vi "SetAttributeViString_SA-Gating_Sweep.vi"(7 "AttributeValue":string, 8 "error in (no error)":errorcluster {"code" format="%.0x"}, 9 "AttributeID":u32(ring)=1250201 items=["ACTIVE_MARKER"=1250201, "DISPLAY_TEXT"=1150119, "INPUT_RF_CORRECTION_COMMENT"=1150737, "INPUT_RF_CORRECTION_DESCRIPTION"=1150738, "IVILXISYNC_ARM_SOURCE_EVENTID"=1950012, "IVILXISYNC_ARM_SOURCE_FILTER"=1950013, "IVILXISYNC_EVENT_DESTINATION_PATH"=1950029, "IVILXISYNC_EVENT_SOURCE"=1950032, "IVILXISYNC_TRIGGER_SOURCE_EVENTID"=1950026, "IVILXISYNC_TRIGGER_SOURCE_FILTER"=1950027, "IVILXISYNC_TRIGGER_SOURCE"=1950022, "MARKER_TRACE"=1250209, "SA_ACP_DISPLAY_TEXT"=1150150, "SA_BURSTPOWER_DISPLAY_TEXT"=1150213, "SA_CHANNELPOWER_DISPLAY_TEXT"=1150305, "SA_LIMIT_COMMENT"=1150618, "SA_OCCUPIEDBANDWIDTH_DISPLAY_TEXT"=1150311, "SA_POWERSTATISTICS_DISPLAY_TEXT"=1150339, "SA_SEMASK_DISPLAY_TEXT"=1150387, "SA_SOURCE_ADDRESS"=1150800, "STATETRIGGER_EVENT_ID"=1150161, "STATETRIGGER_FILTER"=1150162, "STATETRIGGER_STATE_LOCATION"=1150163, "SYSTEM_DATE"=1150172, "SYSTEM_TIME"=1150174, "TEXT"=1150431], 10 "RepCapIdentifier":string, 11 "instrument handle":refnum<k15>) -> (0 "error out":errorcluster {"code" format="%.0x"}, 3 "instrument handle out":refnum<k15>)   [LabVIEW 2009, in "Keysight XSAn.lvlib"]
doc: "Sets a String attribute from the instrument driver.\nThe following Attributes are supported:\n\nACTIVE_MARKER\nDISPLAY_TEXT\nINPUT_RF_CORRECTION_COMMENT\nINPUT_RF_CORRECTION_DESCRIPTION\nIVILXISYNC_ARM_SOURCE_EVENTID\nIVILXISYNC_ARM_SOURCE_FILTER\nIVILXISYNC_EVENT_DESTINATION_PATH\nIVILXISYNC_EVENT_SOURCE\nIVILXISYNC_TRIGGER_SOURCE_EVENTID\nIVILXISYNC_TRIGGER_SOURCE_FILTER\nIVILXISYNC_TRIGGER_SOURCE\nMARKER_TRACE\nSA_ACP_DISPLAY_TEXT\nSA_BURSTPOWER_DISPLAY_TEXT\nSA_CHANNELPOWER_DISPLAY_TEXT\nSA_LIMIT_COMMENT\nSA_OCCUPIEDBANDWIDTH_DISPLAY_TEXT\nSA_POWERSTATISTICS_DISPLAY_TEXT\nSA_SEMASK_DISPLAY_TEXT\nSA_SOURCE_ADDRESS\nSTATETRIGGER_EVENT_ID\nSTATETRIGGER_FILTER\nSTATETRIGGER_STATE_LOCATION\nSYSTEM_DATE\nSYSTEM_TIME\nTEXT"
uses:
  <instrlib>/Keysight XSAn/Keysight XSAn.lvlib
  AgXSAn.dll
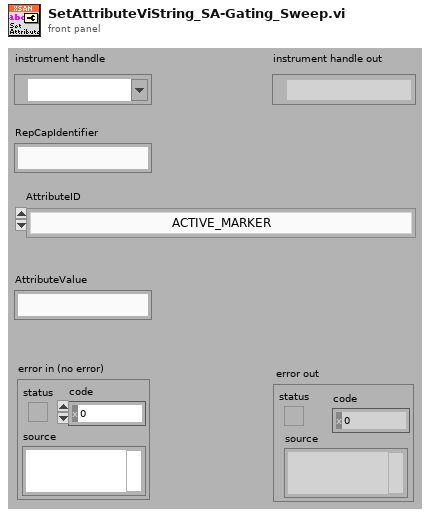
[diagram p1: front panel]
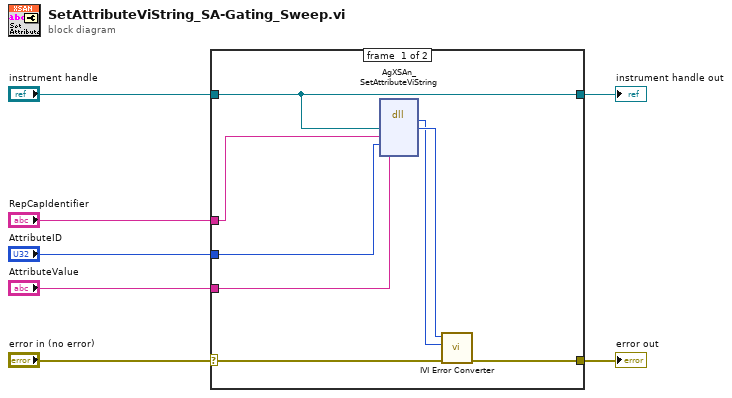
[diagram p0: block diagram]
diagram:
  n1 = case shown="No Error" "error in (no error)" {
    selector: "error in (no error)" -> [w13 w17]
    tunnel: [w12 w17] -> w7
    tunnel: "instrument handle" -> [w8 w16]
    tunnel: "RepCapIdentifier" -> [w11 _]
    tunnel: "AttributeID" -> [w10 _]
    tunnel: "AttributeValue" -> [w9 _]
    tunnel: [w8 w16] -> w1
    frame #0 {
      n2 = dll-call lib="AgXSAn**.dll" fn="AgXSAn_SetAttributeViString"("Vi"=w8, "RepCapIdentifier"=w11, "AttributeID"=w10, "AttributeValue"=w9) -> ("return type"=w14:i32, "Vi"=w15:u32)  [unwired: 6 in, 2 out]
      n3 = call <instrlib>:"IVI Error Converter.vi"("error in (no error)"=w13, "IVI error code (0)"=w14, "instrument handle"=w15) -> ("error out"=w12:errorcluster)  [unwired: 7 in, 1 out]
    }
    frame #1 {
    }
  }
  "error out" <- w7
  "instrument handle out" <- w1
